vi "ex03_operators.vi"() -> ()   [LabVIEW 2019]
panel:
  out "Waveform Chart":dbl(graph)
  out "<0.2":bool
  out "number (0 to 1)":dbl
  out "Numeric":i32
  out ".not. x? 2":bool
  in  "Boolean":bool
  out ".not. x?":bool
  in  "stop":bool
  # "OFF"
  # "ON"
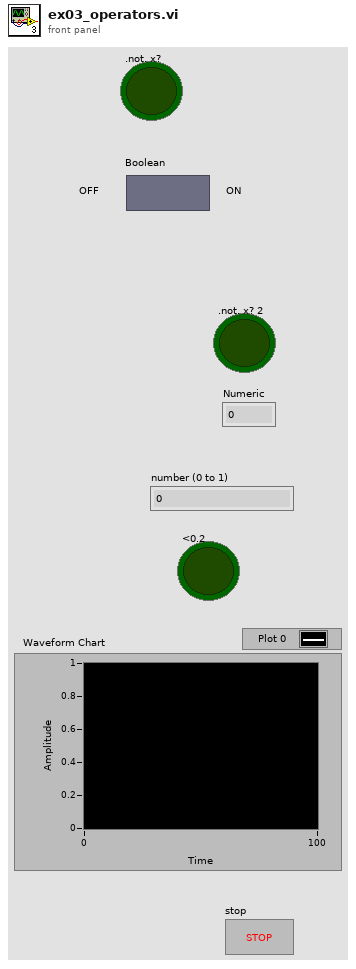
[diagram p1: front panel]
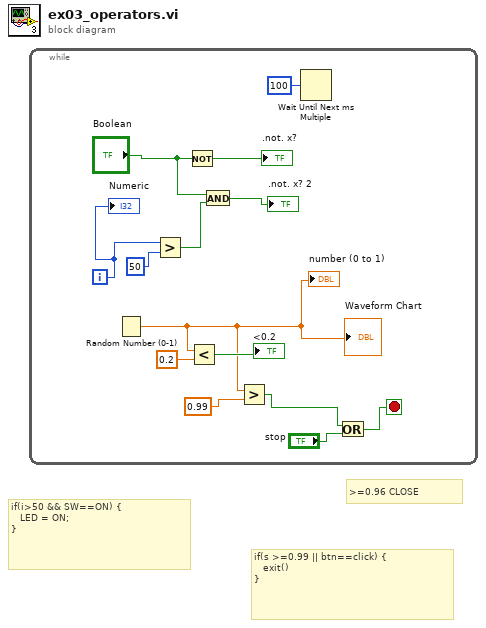
[diagram p0: block diagram]
diagram:
  # "if(s >=0.99 || btn==click) {\n   exit()\n}"
  # ">=0.96 CLOSE"
  # "if(i>50 && SW==ON) {\n   LED = ON;\n}"
  n1 = while {
    i -> [w11]
    stop <- w1 stop-if-true
    n2 = Random Number (0-1)() -> (number: 0 to 1=w5:dbl)
    "number (0 to 1)" <- w5
    "Waveform Chart" <- w5
    n3 = Greater?(x=w11, y=50) -> (0:w9:bool)
    n4 = Not(x="Boolean") -> (.not. x?=→".not. x?":bool)
    n5 = Less?(x=w5, y=0.2) -> (x < y?=→"<0.2":bool)
    n6 = And(x="Boolean", y=w9) -> (x .and. y?=→".not. x? 2":bool)
    n7 = Greater?(x=w5, y=0.99) -> (0:w3:bool)
    n8 = Wait Until Next ms Multiple(millisecond multiple=u32 100) -> ()  [unwired: 1 out]
    n9 = Or(x=w3, y="stop") -> (x .or. y?=w1:bool)
    "Numeric" <- w11
  }
